vi "Intro-ReadRatesFromModules.vi"() -> ()   [LabVIEW 2023]
doc: "This example demonstrates how to get correct values from the initialised and selected SPC modules for different rates like the sync rate, CFD rate, TAC rate as well as ADC rate.\nNote, that the \"rate count time\" parameter is set to 1 second as a default value. This can be changed using the \"SPC_set-parameter.vi\" with keyword \"rate count time\".\n\ninfo@becker-hickl.com"
uses:
  SPC_Wrappers/SPC_Controls/SPCModInfo.ctl
  SPC_Wrappers/SPC_Controls/ModuleType.ctl
  SPC_Wrappers/SPC_Controls/SPC_RatesCluster.ctl
  SPC_Wrappers/SPC_Controls/ModuleTypes.ctl
panel:
  out "SPC_RatesCluster":T1[](array[typedef]) {"Sync" scale=0.0..6000000.0; "ADC" scale=0.0..1000000.0; "TAC" scale=0.0..1000000.0; "CFD" scale=0.0..1000000.0}
  in  "Stop Button":bool
  out "Serial Number":string[](array[string])
  out "Active Module No":i16[](array[numeric])
  out "Used Model Array":T2[](array[typedef]) {"Bus Number" min=-1 max=255 step=1; "Base I/O Addr" format="%.0x"; "Init Status" min=-10 max=0 step=1; "in Use" min=-1 max=1 step=1; "Slot Number" min=-1 max=255 step=1; "Module Type" items=["SPC-600"=600, "SPC-630"=630, "SPC-700"=700, "SPC-730"=730, "SPC-130"=130, "SPC-830"=830, "SPC-140"=140, "SPC-930"=930, "DPC-230"=230, "SPC-150"=150, "SPC-150 N"=151, "SPC-150 NX"=152, "SPC-130 EM"=131, "SPC-130 EMN"=132, "SPC-130IN"=135, "SPC-130INX"=136, "SPC-130INXX"=137, "SPC-160"=160, "SPC-160 X"=161, "SPC-160 PCIE"=162, "SPC-180 N"=180, "SPC-180 NX"=181, "SPC-180 NXX"=182, "SPC-180 N-USB"=185, "SPC-180 NX-USB"=186, "SPC-180 NXX-USB"=187, "SPC-QC-104"=104, "SPC-QC-004"=4, "SPC-QC-106"=106, "DPC-330"=330, "PMS-800"=800, "SPC-590"=590, "Simulation"=-1]}
  # "This example demonstrates how to get correct values from the initialised and selected SPC modules for different rates like the sync rate, CFD rate, TAC rate as well as ADC rate."
  # "(c) 202 Becker & Hickl GmbH\n     All Rights Reserved."
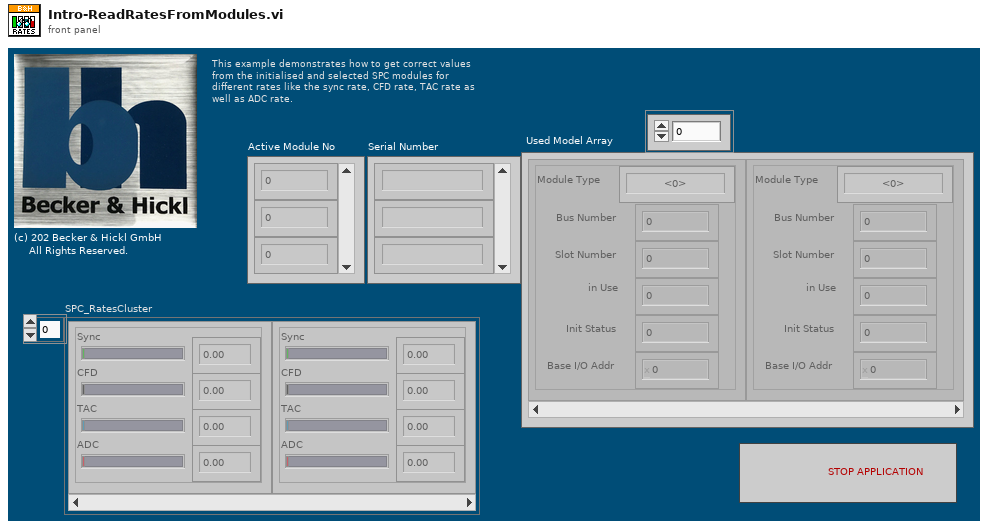
[diagram p1: front panel]
types:
  T1 = typedef "SPC_RatesCluster.ctl" = cluster{"Sync":sgl, "CFD":sgl, "TAC":sgl, "ADC":sgl}
  T2 = typedef "SPCModInfo.ctl" = cluster{"Module Type":T3, "Bus Number":i16, "Slot Number":i16, "in Use":i16, "Init Status":i16, "Base I/O Addr":u16}
  T3 = typedef "ModuleType.ctl" = i16
  T4 = typedef "ModuleTypes.ctl" = i16
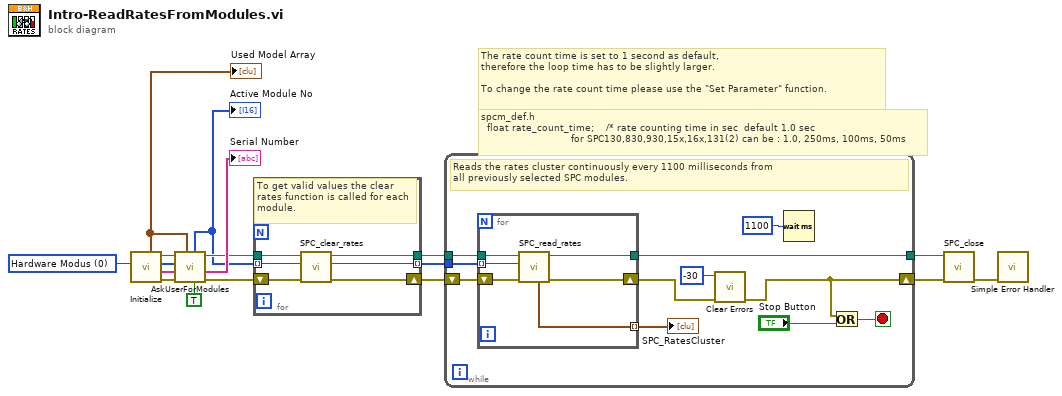
[diagram p0: block diagram]
diagram:
  w9 = T4 0 items=["Hardware Modus"=0, "SPC-600 Simulation"=600, "SPC-630 Simulation"=630, "SPC-700  Simulation"=700, "SPC-730  Simulation"=730, "SPC-130  Simulation"=130, "SPC-830  Simulation"=830, "SPC-140  Simulation"=140, "SPC-930  Simulation"=930, "DPC-230  Simulation"=230, "SPC-150  Simulation"=150, "SPC-150 N  Simulation"=151, "SPC-150 NX  Simulation"=152, "SPC-130 EM  Simulation"=131, "SPC-130 EMN  Simulation"=132, "SPC-160  Simulation"=160, "SPC-160 X  Simulation"=161, "SPC-160 PCIE  Simulation"=162, "DPC-330  Simulation"=330, "DPC 590  Simulation"=590] ("Modul Type to Simulate")
  # "spcm_def.h\n  float rate_count_time;    /* rate counting time in sec  default 1.0 sec\n                              for SPC130,830,930,15x,16x,131(2) can be : 1.0, 250ms, 100ms, 50ms"
  # "The rate count time is set to 1 second as default,\ntherefore the loop time has to be slightly larger.\n\nTo change the rate count time please use the \"Set Parameter\" function."
  n1 = call "Initialize.vi"("Modul Type to Simulate"=w9) -> ("ErrorOut"=w16:errorcluster, "SerialNumbersArray"=w14:string[], "ModuleNoArray"=w15:i16[], "DLL Path"=w17:path, "SPCModulesArray"=w4:T2[])  [unwired: 6 in]
  "Used Model Array" <- w4
  n2 = call "AskUserForModules.vi"("MultiModule"=TRUE, "SPCModulesArray"=w4, "Error In"=w16, "Serial Number"=w14, "ModuleNoArray"=w15, "DLL Path"=w17) -> ("Error Out"=w8:errorcluster, "ActiveSerialNumbers"=→"Serial Number":string[], "DLL Path"=w7:path, "ActiveModuleNo"=w3:i16[])  [unwired: 1 in, 1 out]
  "Active Module No" <- w3
  n3 = for {
    tunnel: w3 -> [w21] mode=indexing
    shift-right: [w20] -> w6
    shift-left: w8 -> [w23]
    tunnel: [w18] -> w2 mode=indexing
    tunnel: w7 -> [w22]
    tunnel: [w19] -> w5
    # "To get valid values the clear\nrates function is called for each module."
    n4 = call "SPC_clear_rates.vi"("Error In"=w23, "Module no"=w21, "DLL Path"=w22) -> ("Error Out"=w20:errorcluster, "Module  No"=w18:i16, "DLL Path"=w19:path)  [unwired: 6 in]
  }
  n5 = while {
    shift-right: [w24] -> w10
    shift-left: w6 -> [w33]
    tunnel: w2 -> [w25]
    tunnel: w5 -> [w34]
    tunnel: [w32] -> w11
    stop <- w28 stop-if-true
    # "Reads the rates cluster continuously every 1100 milliseconds from \nall previously selected SPC modules."
    n6 = for {
      shift-right: [w37] -> w27
      shift-left: w33 -> [w39]
      tunnel: [w36] -> w30 mode=indexing
      tunnel: w25 -> [w35] mode=indexing
      tunnel: w34 -> [w40]
      tunnel: [w38] -> w32
      n7 = call "SPC_read_rates.vi"("Error In"=w39, "Module No"=w35, "DLL Path"=w40) -> ("Error Out"=w37:errorcluster, "DLL Path"=w38:path, "SPC_RatesCluster"=w36:T1)  [unwired: 5 in, 1 out]
    }
    "SPC_RatesCluster" <- w30
    n8 = call <vilib>:"Clear Errors.vi"("error in (no error)"=w27, "specific error code to clear (0: all)"=-30) -> ("error out"=w24:errorcluster)  [unwired: 4 in, 1 out]
    n9 = Wait (ms)(milliseconds to wait=u32 1100) -> ()  [unwired: 1 out]
    n10 = Or(x=w24, y="Stop Button") -> (x .or. y?=w28:bool)
  }
  n11 = call "SPC_close.vi"("Error In"=w10, "DLL Path"=w11) -> ("Error Out"=w13:errorcluster)  [unwired: 8 in, 1 out]
  n12 = call <vilib>:"Simple Error Handler.vi"("error in (no error)"=w13) -> ()  [unwired: 4 in, 5 out]
